vi "Connection State Callback.vi"(7 "Owner":refnum<class>, 8 "error in (no error)":errorcluster, 9 "Context":variant, 10 "Connection State":T1, 11 "Connection":refnum<class "Connection.lvclass">) -> (0 "error out":errorcluster)   [LabVIEW 2020, in "Terminal.lvlib" / "Terminal.lvclass"]
uses:
  Terminal.lvclass
  <vilib>/IlluminatedG/lv-stream/Connection/Connection.lvclass
  <vilib>/IlluminatedG/lv-stream/Connection State.ctl
  Terminal.lvclass/Terminal.ctl
  <vilib>/IlluminatedG/lv-stream/Stream.lvlib
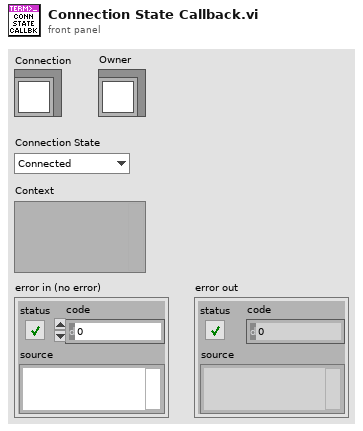
[diagram p1: front panel]
types:
  T1 = typedef "Stream.lvlib/Connection State.ctl" = enum16{"Connected", "Disconnected"}
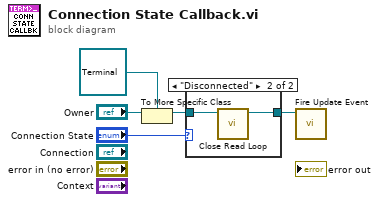
[diagram p0: block diagram]
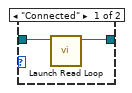
[diagram p2: hidden frame]
diagram:
  n1 = To More Specific Class(target class=refnum<class "Terminal.lvclass"> refnum ("Terminal.lvlib:Terminal.lvclass"), reference="Owner") -> (specific class reference=w2:refnum<class "Terminal.lvclass">)  [unwired: 1 in, 1 out]
  n2 = case shown="\"Disconnected\"" "Connection State" {
    tunnel: w2 -> [w7 w9]
    tunnel: [w6 w8] -> w1
    frame "Connected" {
      n3 = call "Launch Read Loop.vi"("Terminal in"=w7) -> ("Terminal out"=w6:refnum<class "Terminal.lvclass">)  [unwired: 9 in, 1 out]
    }
    frame "Disconnected" {
      n4 = call "Close Read Loop.vi"("Terminal in"=w9) -> ("Terminal out"=w8:refnum<class "Terminal.lvclass">)  [unwired: 9 in, 1 out]
    }
  }
  n5 = call "Fire Update Event.vi"("Terminal in"=w1) -> ()  [unwired: 9 in, 2 out]
